vi "auto_focus.vi"(6 "counts":refnum<vi>, 8 "dwell_time_ms":dbl=100.0, 9 "q_steps":i32=100, 10 "z_end":dbl=100.0, 11 "z_start":dbl) -> (2 "focus_data":cluster{"z_values":dbl[], dbl[]}, 3 "z_focus":dbl)   [LabVIEW 2018]
uses:
  <vilib>/Analysis/1siggen.llb/Ramp Pattern by Samples.vi
  <vilib>/Analysis/NI_AALBase.lvlib
panel:
  # "Distances are measured in um."
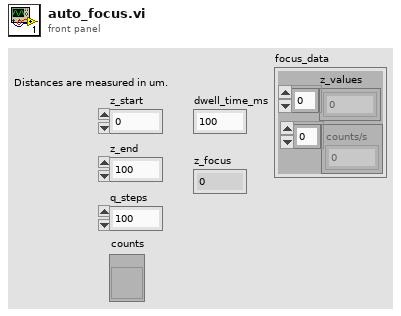
[diagram p1: front panel]
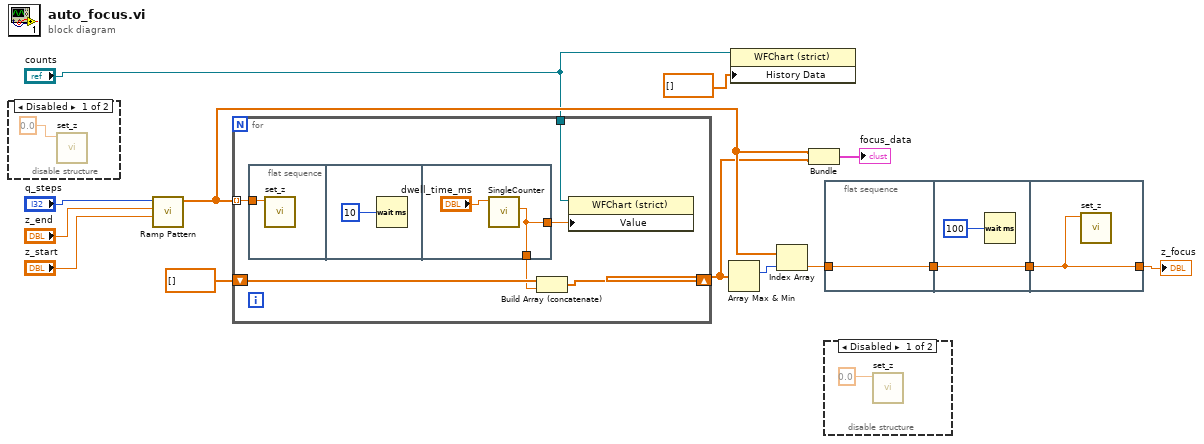
[diagram p0: block diagram]
diagram:
  n1 = disable-structure shown="Disabled" {
    frame Disabled {
      n2 = call "set_z.vi"("z_value_um"=0.0 ("z_value")) -> ()  [unwired: 10 in, 1 out]
    }
    frame Enabled {
    }
  }
  n3 = call-poly <vilib>:"Ramp Pattern.vi"("start"="z_start", "end"="z_end", "samples"="q_steps") -> ("Ramp Pattern"=w5:dbl[])  [unwired: 7 in, 1 out]
  n4 = for {
    tunnel: w5 -> [w21] mode=indexing
    shift-right: [w18] -> w4
    shift-left: dbl[] [] -> [w20]
    tunnel: "counts" -> [w17]
    n5 = flat-sequence {
      tunnel: w21 -> [w22]
      tunnel: [w24] -> w19
      tunnel: [w24] -> w16
      frame #0 {
        n6 = call "set_z.vi"("z_value_um"=w22) -> ()  [unwired: 10 in, 1 out]
      }
      frame #1 {
        n7 = Wait (ms)(milliseconds to wait=u32 10) -> ()  [unwired: 1 out]
      }
      frame #2 {
        n8 = call "SingleCounter.vi"("Dwell_time_ms"="dwell_time_ms") -> ("counts/s"=w24:dbl)  [unwired: 8 in, 2 out]
      }
    }
    n9 = Build Array (concatenate)(w20, w19) -> (w18:dbl[])
    n10 = property class="WFChart (strict)"(reference=w17, "Value"=w16) -> ()  [unwired: 1 in, 2 out]
  }
  n11 = Array Max & Min(array=w4) -> (max index (indices)=w11:i32)  [unwired: 3 out]
  n12 = property class="WFChart (strict)"(reference="counts", "History Data"=dbl[] []) -> ()  [unwired: 1 in, 2 out]
  n13 = Index Array(array=w5, index=w11) -> (element=w7:dbl)
  n14 = Bundle("Ramp Pattern"=w5, w4) -> (→"focus_data":cluster{"Ramp Pattern":dbl[], dbl[]})  [unwired: 1 in]
  n15 = flat-sequence {
    tunnel: [w26] -> w8
    tunnel: w7 -> [w26]
    tunnel: [w27] -> w9
    tunnel: w8 -> [w27]
    tunnel: w9 -> [w29]
    tunnel: [w29] -> w6
    frame #0 {
    }
    frame #1 {
      n16 = Wait (ms)(milliseconds to wait=u32 100) -> ()  [unwired: 1 out]
    }
    frame #2 {
      n17 = call "set_z.vi"("z_value_um"=w29) -> ()  [unwired: 10 in, 1 out]
    }
  }
  n18 = disable-structure shown="Disabled" {
    frame Disabled {
      n19 = call "set_z.vi"("z_value_um"=0.0 ("z_value")) -> ()  [unwired: 10 in, 1 out]
    }
    frame Enabled {
    }
  }
  "z_focus" <- w6
